vi "Read Measurement Units.vi"(8 "error in":errorcluster, 11 "thermocouple channel in":refnum<class "Thermocouple Channel.lvclass">) -> (0 "error out":errorcluster, 2 "measurement units":T1, 3 "thermocouple channel out":refnum<class "Thermocouple Channel.lvclass">)   [LabVIEW 2017, in "Scan Engine Scripting.lvlib" / "Thermocouple Channel.lvclass"]
doc: "Reads the measurement units from the private data of the channel."
uses:
  Thermocouple Channel.lvclass
  Measurement Units.ctl
  Thermocouple Channel.lvclass/Thermocouple Channel.ctl
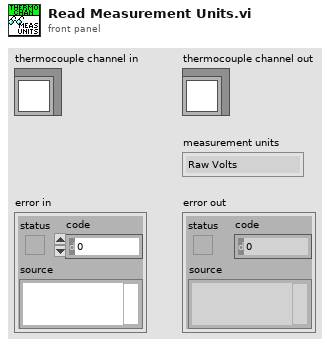
[diagram p1: front panel]
types:
  T1 = typedef "Scan Engine Scripting.lvlib/Thermocouple Channel.lvclass/Measurement Units.ctl" = enum16{"Raw Volts", "Degrees Kelvin", "Degrees Celsius", "Degrees Fahrenheit", "Degrees Rankine"}
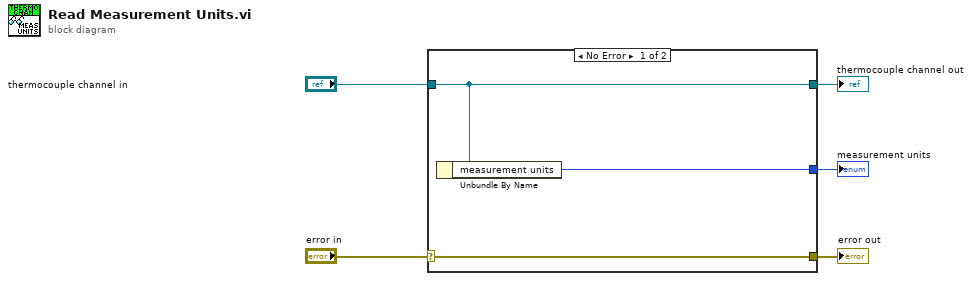
[diagram p0: block diagram]
diagram:
  n1 = case shown="No Error" "error in" {
    selector: "error in" -> [w8 w9]
    tunnel: [w8 w9] -> w4
    tunnel: [w7 w10] -> w2
    tunnel: "thermocouple channel in" -> [w7 w10]
    tunnel: [w6 _] -> w1
    frame No Error {
      n2 = Unbundle By Name(w7) -> ("measurement units"=w6:T1)
    }
    frame Error {
    }
  }
  "error out" <- w4
  "thermocouple channel out" <- w2
  "measurement units" <- w1
